vi "GitFilteredLog.vi"(8 "error in (no error)":errorcluster, 9 "Directory":path=path "", 10 "Filter":string, 11 "Git exec":string="git") -> (0 "error out":errorcluster, 1 "Directory out":path, 2 "Detail Array":string[][](array[string]), 3 "Git exec out":string="git", 4 "Number Matched":i32)   [LabVIEW 2013]
uses:
  <vilib>/Utility/error.llb/whitespace.ctl
  GitCommitCluster/CommitCluster.ctl
  GitCmd.vi
  <vilib>/dlg_ctls.llb/Space Constant.vi
  <vilib>/Utility/error.llb/General Error Handler.vi
  GitUtils/PathtoDirPath.vi
  <vilib>/Platform/system.llb/System Exec.vi
  <vilib>/Utility/error.llb/Error Cluster From Error Code.vi
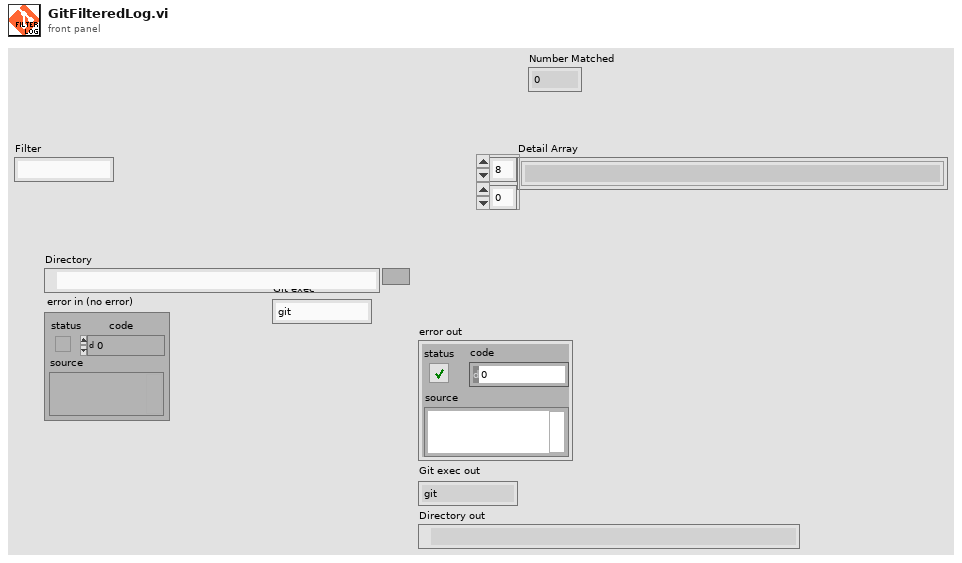
[diagram p1: front panel]
types:
  T1 = typedef "whitespace.ctl" = u16
  T2 = typedef "CommitCluster.ctl" = cluster{"Hash":string, "Date":string, "Name":string}
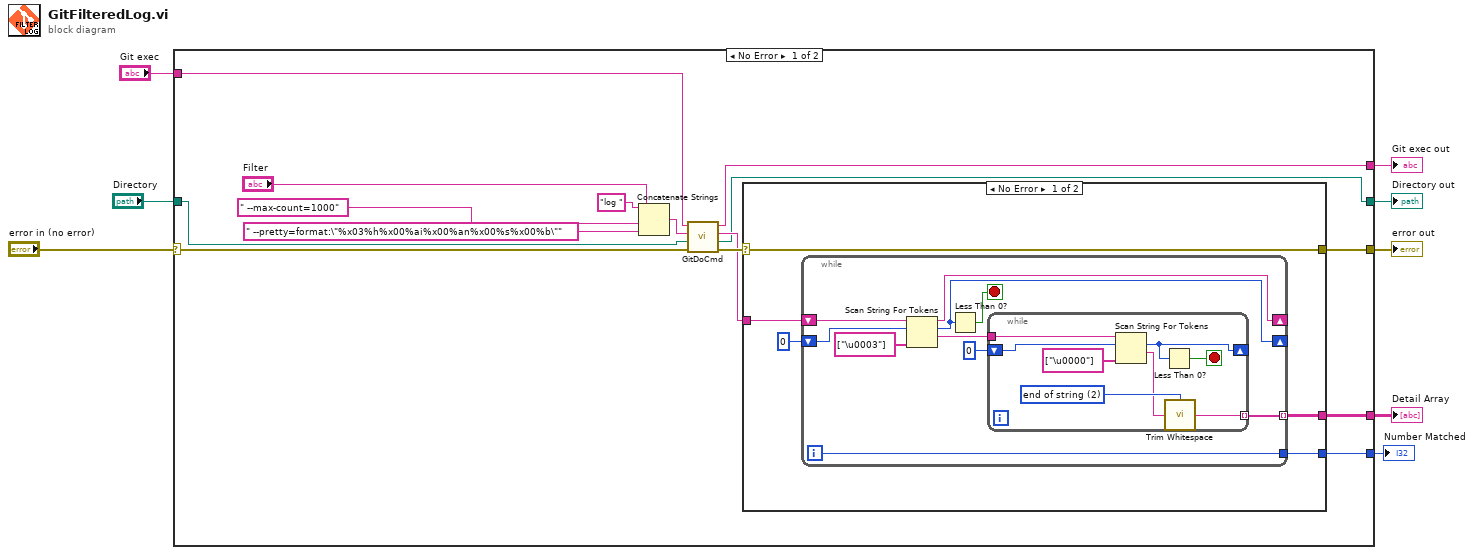
[diagram p0: block diagram]
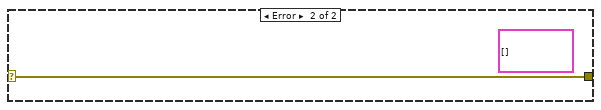
[diagram p2: hidden frame]
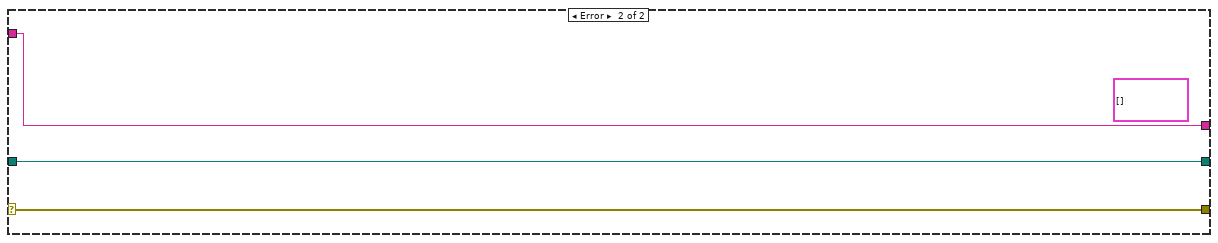
[diagram p3: hidden frame]
diagram:
  n1 = case shown="No Error" "error in (no error)" {
    selector: "error in (no error)" -> [w20 w50]
    tunnel: "Git exec" -> [w17 w49]
    tunnel: "Directory" -> [w13 w48]
    tunnel: [w21 w50] -> w6
    tunnel: [w16 w49] -> w4
    tunnel: [w14 w48] -> w3
    tunnel: [w12 _] -> w2
    tunnel: [w9 _] -> w1
    frame No Error {
      n2 = Concatenate Strings("log " ("string"), "Filter", " --max-count=1000" ("string"), " --pretty=format:\"%x03%h%x00%ai%x00%an%x00%s%x00%b\"" ("string")) -> (w18:string)
      n3 = call "GitDoCmd.vi"("error in (no error)"=w20, "Working Path"=w13, "Git command"=w18, "Git exec"=w17) -> ("error out"=w19:errorcluster, "Working Path out"=w14:path, "Returned stdout"=w15:string, "Git exec out"=w16:string)  [unwired: 3 in]
      n4 = case shown="No Error" w19 {
        selector: w19 -> [w28 w47]
        tunnel: w15 -> [w27 _]
        tunnel: [w28 w47] -> w21
        tunnel: [w26 _] -> w12
        tunnel: [w24 _] -> w9
        frame No Error {
          n5 = while {
            shift-right: [w36] -> _
            shift-left: w27 -> [w38]
            tunnel: [w31] -> w26 mode=indexing
            shift-right: [w33] -> _
            shift-left: 0 ("offset past token") -> [w35]
            tunnel: [w29] -> w24
            i -> [w29]
            stop <- w34 stop-if-true
            n6 = Scan String For Tokens(6:string[] ["\u0003"] ("delimiters (\\s,\\t,\\r,\\n)"), 8:w35, 9:w38) -> (1:w32:string, 2:w33:i32, 3:w36:string)  [unwired: 3 in, 1 out]
            n7 = Less Than 0?(x=w33) -> (x < 0?=w34:bool)
            n8 = while {
              tunnel: w32 -> [w44]
              tunnel: [w39] -> w31 mode=indexing
              shift-right: [w43] -> _
              shift-left: 0 ("offset past token") -> [w42]
              stop <- w45 stop-if-true
              w41 = T1 2 items=["both", "start of string", "end of string"] ("location (both)")
              n9 = Scan String For Tokens(6:string[] ["\u0000"] ("delimiters (\\s,\\t,\\r,\\n)"), 8:w42, 9:w44) -> (1:w40:string, 2:w43:i32)  [unwired: 3 in, 2 out]
              n10 = Less Than 0?(x=w43) -> (x < 0?=w45:bool)
              n11 = call <vilib>:"Trim Whitespace.vi"("string"=w40, "location (both)"=w41) -> ("trimmed string"=w39:string)
            }
          }
        }
        frame Error {
          (unwired) T2[] [] ("Array")
        }
      }
    }
    frame Error {
      (unwired) T2[] [] ("Array")
    }
  }
  "error out" <- w6
  "Git exec out" <- w4
  "Directory out" <- w3
  "Detail Array" <- w2
  "Number Matched" <- w1
